vi "LAUNCHER.vi"() -> ()   [LabVIEW 2020]
uses:
  UI Actor/UI Actor.lvclass
  C:/Program Files/National Instruments/LabVIEW 2020/vi.lib/ActorFramework/Actor/Actor.lvclass
  Implementacion/NXP/NXP.lvclass
  C:/Users/Ceci Saldivar/Documents/ceci/7mo semestre/Henry/ya ultimo proyecto alv ptm/Proyecto-final-2000/Abstract/Serial Device/Serial Device.lvclass
  Implementacion/Simulated/Simulated.lvclass
  Implementacion/Arduino/Arduino.lvclass
  UI Actor/UI Actor.lvclass/UI Actor.ctl
  UI Actor/Write Serial Device.lvclass.vi
  UI Actor/Write VISA resource name.vi
  <vilib>/ActorFramework/Actor/Actor.lvclass
panel:
  in  "Text Ring":u16(ring) items=["NXP", "Arduino", "Simulado"]
  in  "COM Port":refnum<visa-resource-name>
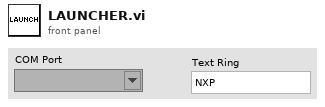
[diagram p1: front panel]
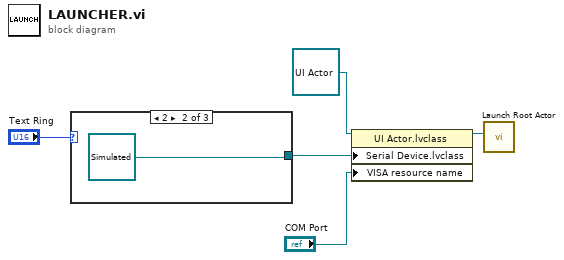
[diagram p0: block diagram]
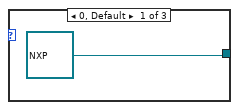
[diagram p2: hidden frame]
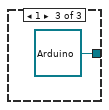
[diagram p3: hidden frame]
diagram:
  n1 = case shown="2" "Text Ring" {
    tunnel: [refnum<class "NXP.lvclass"> refnum ("NXP.lvclass") refnum<class "Simulated.lvclass"> refnum ("Simulated.lvclass") refnum<class "Arduino.lvclass"> refnum ("Arduino.lvclass")] -> w2
    frame 0, Default {
    }
    frame 2 {
    }
    frame 1 {
    }
  }
  n2 = property class="UI Actor.lvclass"(reference=refnum<class "UI Actor.lvclass"> refnum ("UI Actor.lvlib:UI Actor.lvclass"), "Serial Device.lvclass"=w2, "VISA resource name"="COM Port") -> (reference out=w1:refnum<class "UI Actor.lvclass">)  [unwired: 1 in, 1 out]
  n3 = call <vilib>:"Launch Root Actor.vi"("Actor"=w1) -> ()  [unwired: 9 in, 2 out]
